vi "PAST_5_DAY_GRAPH.vi"(8 "error in (no error) 2":errorcluster, 11 "5 date":string[](array[string])) -> (0 "error out":errorcluster, 3 "Array 2":timestamp[](array[timestamp]))   [LabVIEW 2017]
uses:
  <vilib>/Utility/miscctls.llb/LVDateTimeRec.ctl
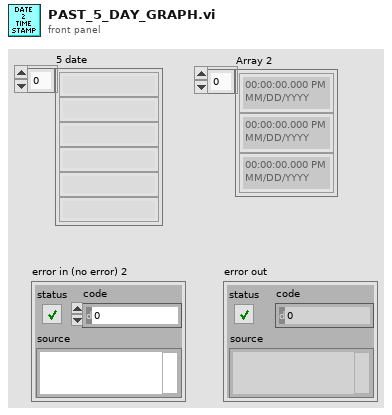
[diagram p1: front panel]
types:
  T1 = typedef "LVDateTimeRec.ctl" = cluster{"fractional second":dbl, "second":i32, "minute":i32, "hour":i32, "day of month":i32, "month":i32, "year":i32, "day of week":i32, "day of year":i32, "DST":i32}
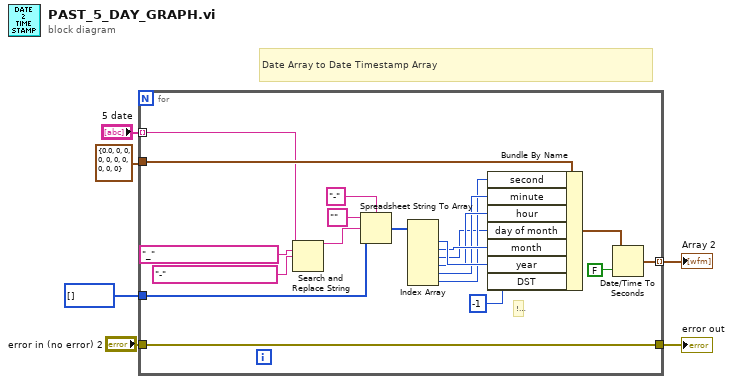
[diagram p0: block diagram]
diagram:
  # "Date Array to Date Timestamp Array"
  n1 = for {
    tunnel: T1 {"fractional second"=0.0, "second"=0, "minute"=0, "hour"=0, "day of month"=0, "month"=0, "year"=0, "day of week"=0, "day of year"=0, "DST"=0} ("Datum/Zeit") -> [w26]
    tunnel: i32[] [] -> [w10]
    tunnel: "5 date" -> [w9] mode=indexing
    tunnel: "error in (no error) 2" -> [w8]
    tunnel: [w8] -> w1
    tunnel: [w7] -> w6 mode=indexing
    # "!!"
    n2 = Search and Replace String(input string=w9, search string="_" ("Such-String"), replace string="-" ("Ersetzungs-String (\"\")")) -> (result string=w21:string)  [unwired: 5 in, 3 out]
    n3 = Spreadsheet String To Array(delimiter (Tab)="-" ("Tabellen-String"), format string="" ("Format-String"), spreadsheet string=w21, array type (2D Dbl)=w10) -> (array=w20:i32[])
    n4 = Index Array(array=w20) -> (element #1=w19:i32, element #2=w18:i32, element #3=w14:i32, element #4=w17:i32, element #5=w16:i32, element #6=w15:i32)  [unwired: 6 in]
    n5 = Bundle By Name(cluster=w26, "second"=w15, "minute"=w16, "hour"=w17, "day of month"=w14, "month"=w18, "year"=w19, "DST"=-1) -> (w12:T1)
    n6 = Date/Time To Seconds(1:FALSE ("Weltzeit (F)"), 2:w12) -> (0:w7:timestamp)
  }
  "Array 2" <- w6
  "error out" <- w1
